vi "Image Display Mousewheel Zoom.vi"() -> ()   [LabVIEW 2015]
uses:
  <vilib>/Utility/miscctls.llb/LVPointTypeDef.ctl
  <vilib>/vision/NI_Vision_Development_Module.lvlib
panel:
  in  "Cancel Button":bool
  out "Image":T1(plugin-control)
  in  "File Path Control":path
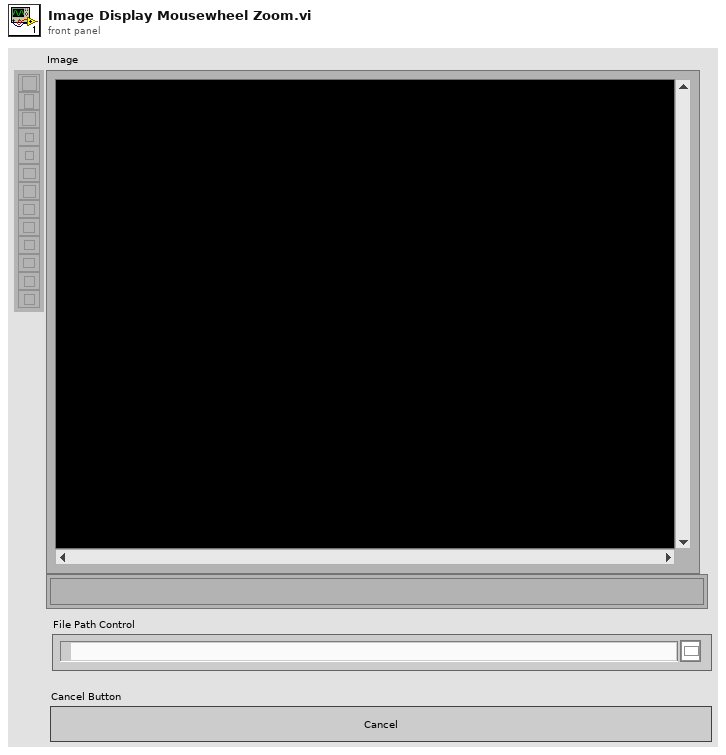
[diagram p1: front panel]
types:
  T1 = typedef "IMAQ Image.ctl" = refnum<image>
  T2 = typedef "Image Type" = u32
  T3 = typedef "LVPointTypeDef.ctl" = cluster{"Horizontal":i16, "Vertical":i16}
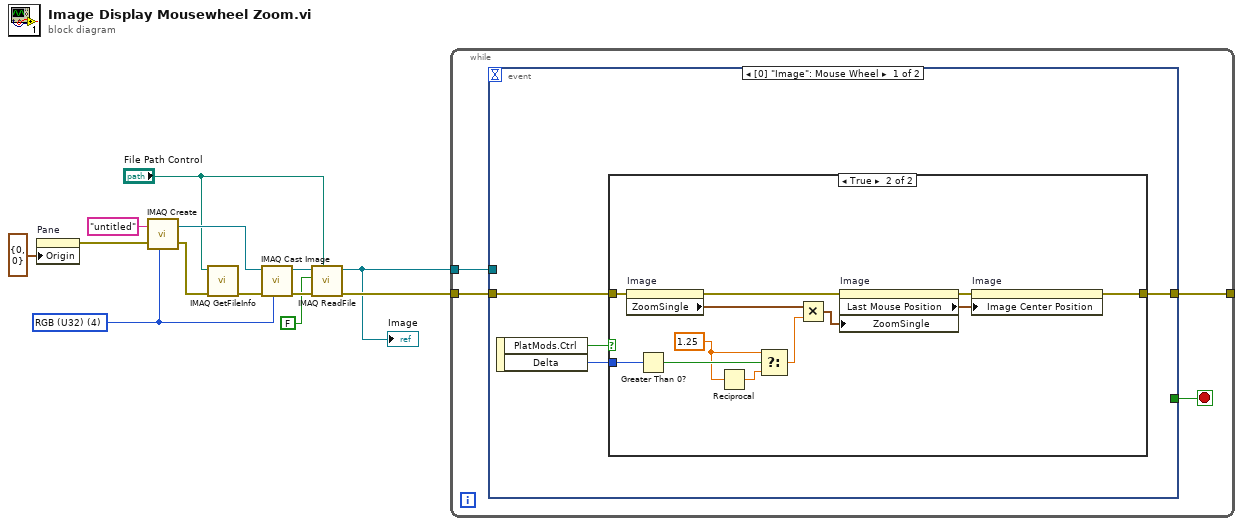
[diagram p0: block diagram]
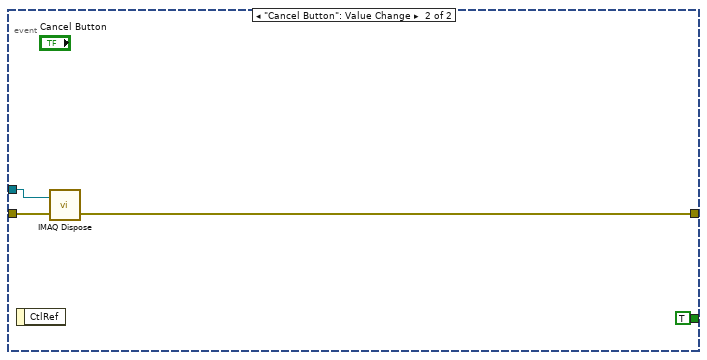
[diagram p3: hidden frame]
diagram:
  w1 = T2 4 items=["Grayscale (U8)", "Grayscale (I16)", "Grayscale (SGL)", "Complex (CSG)", "RGB (U32)", "HSL (U32)", "RGB (U64)", "Grayscale (U16)"] ("Image Type")
  n1 = property on="Pane" class="Pane"("Origin"=T3 {"Horizontal"=0, "Vertical"=0}) -> (error out=w3:errorcluster)  [unwired: 2 in, 1 out]
  n2 = call "IMAQ Create"("Image Name"="untitled", "Image Type"=w1, "error in (no error)"=w3) -> ("New Image"=w10:T1, "error out"=w12:errorcluster)  [unwired: 2 in]
  n3 = call "IMAQ GetFileInfo"("error in (no error)"=w12, "File Path"="File Path Control") -> ("error out"=w11:errorcluster)  [unwired: 3 in, 6 out]
  n4 = call "IMAQ Cast Image"("Image Type"=w1, "error in (no error)"=w11, "Image Src"=w10) -> ("error out"=w9:errorcluster, "Image Dst Out"=w8:T1)  [unwired: 7 in]
  n5 = call "IMAQ ReadFile"("File Path"="File Path Control", "error in (no error)"=w9, "Load Color Palette? (No)"=FALSE, "Image"=w8) -> ("error out"=w5:errorcluster, "Image Out"=w4:T1)  [unwired: 3 in, 3 out]
  "Image" <- w4
  n6 = while {
    tunnel: w4 -> [w17]
    tunnel: w5 -> [w16]
    tunnel: [w15] -> _
    stop <- w14 stop-if-true
    n7 = event shown="[0] \"Image\": Mouse Wheel" {
      selector: _ -> [_ _]
      dyn-events: _ -> [_ _]
      timeout: _ -> [_ _]
      tunnel: w17 -> [_ w37]
      tunnel: w16 -> [w21 w38]
      tunnel: [w19 w36] -> w15
      tunnel: [_ TRUE] -> w14
      event "Image": Mouse Wheel {
        n8 = event-data() -> ("PlatMods.Ctrl"=w18:bool, "Delta"=w20:i32)  [unwired: 1 in]
        n9 = case shown="True" w18 {
          tunnel: w21 -> [w22 w34]
          tunnel: w20 -> [_ w33]
          tunnel: [w22 w23] -> w19
          frame False {
          }
          frame True {
            w30 = 1.25
            n10 = property on="Image" class="ImageControl"(error in=w34) -> (error out=w27:errorcluster, "ZoomSingle"=w28:cluster{"X":sgl, "Y":sgl})  [unwired: 1 in, 1 out]
            n11 = Greater Than 0?(x=w33) -> (x > 0?=w32:bool)
            n12 = Reciprocal(x=w30) -> (1/x=w31:dbl)
            n13 = Select(t=w30, s=w32, f=w31) -> (s? t:f=w29:dbl)
            n14 = Multiply(x=w28, y=w29) -> (x*y=w26:cluster{"X":dbl, "Y":dbl})
            n15 = property on="Image" class="ImageControl"(error in=w27, "ZoomSingle"=w26) -> (error out=w25:errorcluster, "Last Mouse Position"=w24:cluster{"X":i32, "Y":i32})  [unwired: 1 in, 1 out]
            n16 = property on="Image" class="ImageControl"(error in=w25, "Image Center Position"=w24) -> (error out=w23:errorcluster)  [unwired: 1 in, 1 out]
          }
        }
      }
      event "Cancel Button": Value Change {
        n17 = event-data() -> ()  [unwired: 1 in, 1 out]
        n18 = call "IMAQ Dispose"("Image"=w37, "error in (no error)"=w38) -> ("error out"=w36:errorcluster)  [unwired: 4 in]
      }
    }
  }
